vi "Periodic Tasks.vi"(8 "error in":errorcluster) -> ()   [LabVIEW 2018]
doc: "This VI runs in parallel to other tasks. It can contain as many user-defined periodic loops as you need. These can carry out PID or other sorts of timed response."
uses:
  <vilib>/Rock Robotics/WPI/ThirdParty/Sensors/navX/_Processing Loop/FRIC_navX_Internal_SPI_ProcessingLoop.vi
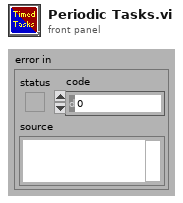
[diagram p1: front panel]
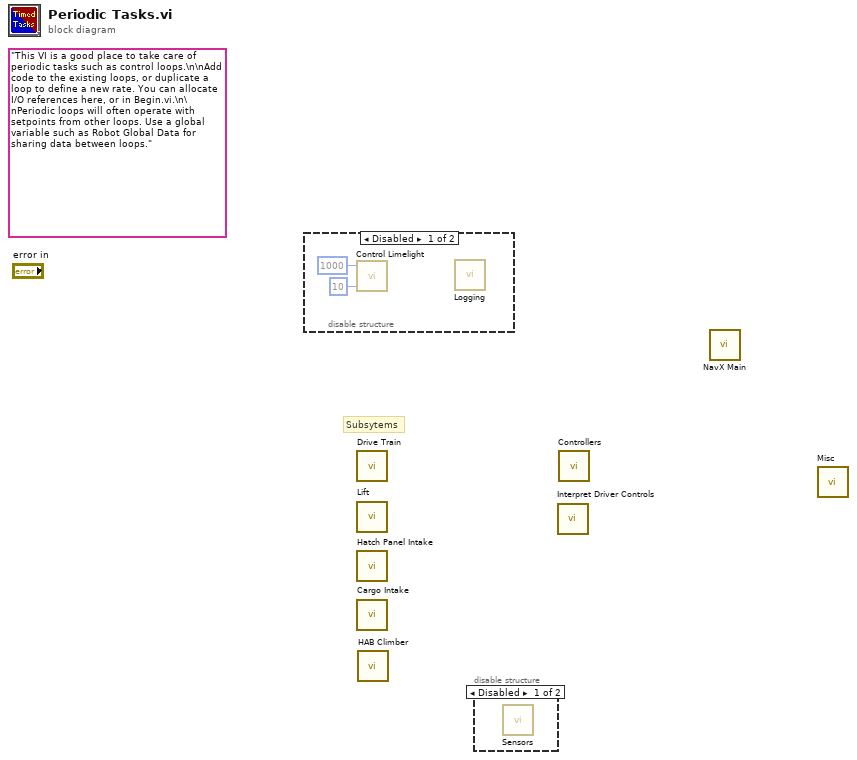
[diagram p0: block diagram]
diagram:
  (unwired) "This VI is a good place to take care of periodic tasks such as control loops.\n\nAdd code to the existing loops, or duplicate a loop to define a new rate. You can allocate I/O references here, or in Begin.vi.\n\nPeriodic loops will often operate with setpoints from other loops. Use a global variable such as Robot Global Data for sharing data between loops."
  # "Subsytems"
  n1 = disable-structure shown="Disabled" {
    frame Disabled {
      n2 = call "Control Limelight.vi"("Read Data Loop Time (ms) (min 10)"=u32 10, "Write Data Loop Time (ms)"=u32 1000) -> ()  [unwired: 1 in]
      n3 = call "Logging.vi"() -> ()  [unwired: 12 in]
    }
    frame Enabled {
    }
  }
  n4 = call "Drive Train.vi"() -> ()  [unwired: 12 in]
  n5 = call "Lift.vi"() -> ()  [unwired: 1 in]
  n6 = call "Hatch Panel Intake.vi"() -> ()  [unwired: 10 in]
  n7 = call "Cargo Intake.vi"() -> ()  [unwired: 12 in]
  n8 = call "HAB Climber.vi"() -> ()  [unwired: 12 in]
  n9 = disable-structure shown="Disabled" {
    frame Disabled {
      n10 = call "Sensors.vi"() -> ()  [unwired: 12 in]
    }
    frame Enabled {
    }
  }
  n11 = call "Interpret Driver Controls.vi"() -> ()  [unwired: 12 in]
  n12 = call "Controllers.vi"() -> ()  [unwired: 12 in]
  n13 = call-poly <vilib>:"NavX Main.vi"() -> ()  [unwired: 12 in]
  n14 = call "Misc.vi"() -> ()  [unwired: 12 in]
